vi "New Client.vi"(4 "write operation timeout":i32=1000, 6 "read operation timeout":i32=1000, 8 "error in (no error)":errorcluster, 9 "connect timeout ms":i32=10000, 11 "WebSocket URL":string) -> (0 "error out":errorcluster, 3 "WebSocket Client out":refnum<class "WebSocket Client.lvclass">)   [LabVIEW 2021, in "WebSockets.lvlib" / "WebSocket Client.lvclass"]
doc: "Opens a conenction and creates a new WebSocket Client using the NI VISA TCP Socket.\nWebSockets 2.0.1.40\nSam Sharp - MediaMongrels Ltd\nCopyright (c) 2019, MediaMongrels Ltd"
uses:
  WebSocket Client.lvclass
  D:/my_projects/projects/Algorithms/Labview/21/WebSockets/WebSockets/WebSocket/WebSocket.lvclass
  Sockets/VISA TCP Socket/VISA TCP.lvclass
  D:/my_projects/projects/Algorithms/Labview/21/WebSockets/Sockets/Socket/Socket.lvclass
  Sockets/VISA TCP Socket/VISA TCP.lvclass/VISA TCP.ctl
  WebSocket/WebSocket.lvclass/WebSocket.ctl
  WebSocket Client.lvclass/WebSocket Client.ctl
  Sockets/VISA TCP Socket/Write port.vi
  Sockets/VISA TCP Socket/Write connect timeout.vi
  WebSocket/Write Socket.vi
  Write URL.vi
  WebSocket/Write read operation timeout.vi
  WebSocket/Write write operation timeout.vi
  <vilib>/Utility/error.llb/Error Cluster From Error Code.vi
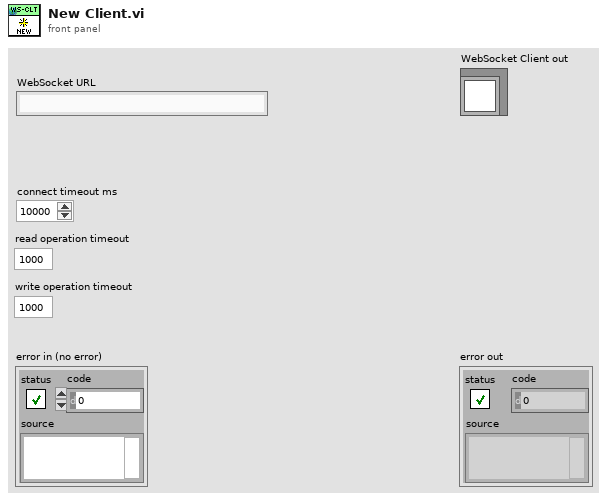
[diagram p1: front panel]
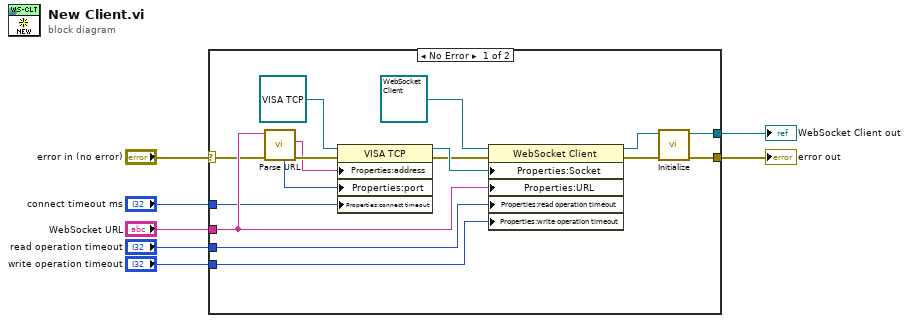
[diagram p0: block diagram]
diagram:
  n1 = case shown="No Error" "error in (no error)" {
    selector: "error in (no error)" -> [w22 w24]
    tunnel: [w10 _] -> w7
    tunnel: [w9 w24] -> w6
    tunnel: "WebSocket URL" -> [w23 _]
    tunnel: "connect timeout ms" -> [w17 _]
    tunnel: "read operation timeout" -> [w14 _]
    tunnel: "write operation timeout" -> [w13 _]
    frame No Error {
      n2 = call "Parse URL.vi"("error in (no error)"=w22, "WebSocket URL"=w23) -> ("error out"=w19:errorcluster, "host"=w8:string, "port"=w18:u16)  [unwired: 5 in, 2 out]
      n3 = property class="VISA TCP"(reference=refnum<class "VISA TCP.lvclass"> refnum ("Sockets:VISA TCP"), error in=w19, "Properties:address"=w8, "Properties:port"=w18, "Properties:connect timeout"=w17) -> (reference out=w16:refnum<class "VISA TCP.lvclass">, error out=w15:errorcluster)
      n4 = property class="WebSocket Client"(reference=refnum<class "WebSocket Client.lvclass"> refnum ("WebSocket Client in"), error in=w15, "Properties:Socket"=w16, "Properties:URL"=w23, "Properties:read operation timeout"=w14, "Properties:write operation timeout"=w13) -> (reference out=w11:refnum<class "WebSocket Client.lvclass">, error out=w12:errorcluster)
      n5 = call "Initialize.vi"("error in (no error)"=w12, "WebSocket Client in"=w11) -> ("error out"=w9:errorcluster, "WebSocket Client out"=w10:refnum<class "WebSocket Client.lvclass">)  [unwired: 8 in]
    }
    frame Error {
    }
  }
  "error out" <- w6
  "WebSocket Client out" <- w7
